vi "(SubVI) fit xyscan-data.vi"(5 "range wanted to fit":dbl, 6 "file path (dialog if empty)":path, 7 "X=T\nY=F":bool=TRUE) -> (1 "Slope (V/um)":dbl)   [LabVIEW 2014]
uses:
  <vilib>/Analysis/6fits.llb/Curve Fitting Criteria.ctl
  <vilib>/Utility/file.llb/Read From Spreadsheet File (DBL).vi
  <vilib>/Analysis/polynomials.llb/Scalar Polynomial Evaluation (DBL).vi
  <vilib>/Analysis/NI_AALPro.lvlib
panel:
  out "Radius for fit-plot":dbl[](array[numeric])
  out "Fit QPD":dbl[](array[numeric])
  out "Aligned QPD (V)":dbl[](array[numeric])
  out "Cut QPD signal (V)":dbl[](array[numeric])
  out "Cut Bead radius (nm)":dbl[](array[numeric])
  out "Bead radius (nm)":dbl[](array[numeric])
  out "Stage":dbl[](array[numeric])
  out "QPD":dbl[](array[numeric])
  out "Polynomial Coefficients":dbl[](array[numeric])
  out "XY Graph":cluster{"all rows":dbl[], "all rows":dbl[]}[](graph)
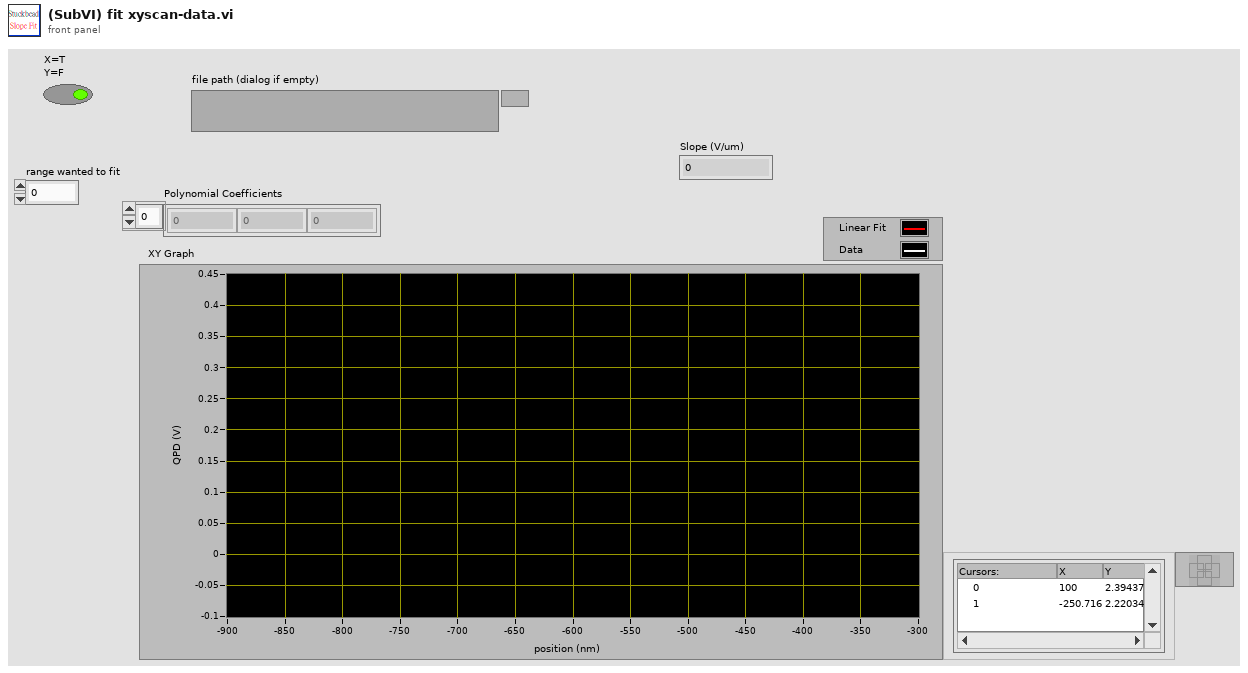
[diagram p1: front panel]
types:
  T1 = typedef "NI_AALPro.lvlib/Curve Fitting Criteria.ctl" = u16
  T2 = cluster{"Bead radius (nm)":dbl[], "Aligned QPD (V)":dbl[]}
  T3 = cluster{"Bead radius (nm)":dbl[], "Aligned QPD (V)":dbl[]}[]
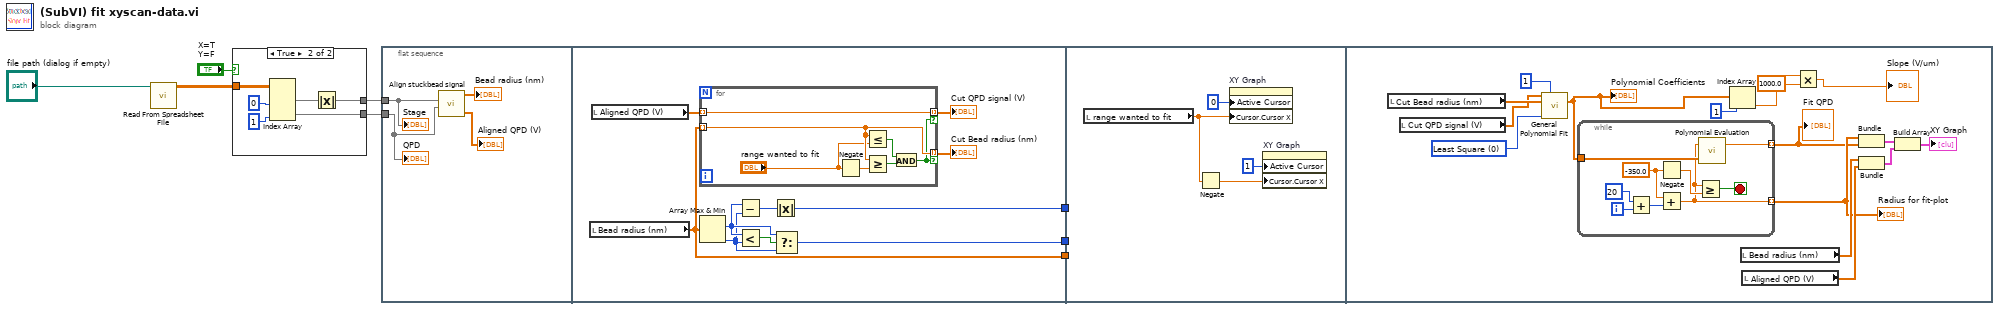
[diagram p0: block diagram]
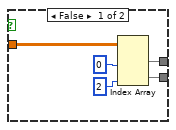
[diagram p2: hidden frame]
diagram:
  n1 = call-poly <vilib>:"Read From Spreadsheet File.vi"("file path (dialog if empty)"="file path (dialog if empty)") -> ("all rows"=w8:dbl[][])  [unwired: 6 in, 4 out]
  n2 = case shown="True" "X=T\nY=F" {
    tunnel: w8 -> [w11 w19]
    tunnel: [w10 w14] -> w6
    tunnel: [w9 w16] -> w5
    frame False {
      n3 = Index Array(array=w11, index (col) #1=0 ("disabled index (col)"), index (col) #2=2 ("index (col)")) -> (element #1=w10:dbl[], element #2=w9:dbl[])  [unwired: 2 in]
    }
    frame True {
      n4 = Index Array(array=w19, index (col) #1=0 ("disabled index (col)"), index (col) #2=1 ("index (col)")) -> (element #1=w15:dbl[], element #2=w16:dbl[])  [unwired: 2 in]
      n5 = Absolute Value(x=w15) -> (abs(x)=w14:dbl[])
    }
  }
  n6 = flat-sequence {
    tunnel: w5 -> [w22]
    tunnel: w6 -> [w23]
    tunnel: [w26] -> w4
    tunnel: [w32] -> w3
    tunnel: [w28] -> w2
    tunnel: w4 -> [_]
    tunnel: w3 -> [_]
    tunnel: w2 -> [_]
    frame #0 {
      n7 = call "Align stuckbead signal.vi"("stuckbstuck QPD (V)"=w22, "Stage (um)"=w23) -> ("Aligned QPD (V)"=→"Aligned QPD (V)":dbl[], "Bead radius (nm)"=→"Bead radius (nm)":dbl[])  [unwired: 3 in]
      "Stage" <- w23
      "QPD" <- w22
    }
    frame #1 {
      n8 = local read "Bead radius (nm)"() -> (w26:dbl[])
      n9 = local read "Aligned QPD (V)"() -> (w27:dbl[])
      n10 = for {
        tunnel: w27 -> [w40] mode=indexing
        tunnel: [w40] -> w24 mode=indexing if=w34
        tunnel: w26 -> [w38] mode=indexing
        tunnel: [w38] -> w25 mode=indexing if=w34
        n11 = Negate(x="range wanted to fit") -> (-x=w39:dbl)
        n12 = Less Or Equal?(x=w38, y="range wanted to fit") -> (x <= y?=w36:bool)
        n13 = Greater Or Equal?(x=w38, y=w39) -> (x >= y?=w35:bool)
        n14 = And(x=w36, y=w35) -> (x .and. y?=w34:bool)
      }
      "Cut Bead radius (nm)" <- w25
      "Cut QPD signal (V)" <- w24
      n15 = Array Max & Min(array=w26) -> (max index (indices)=w30:i32, min index (indices)=w29:i32)  [unwired: 2 out]
      n16 = Subtract(x=w30, y=w29) -> (x-y=w33:i32)
      n17 = Less?(x=w30, y=w29) -> (x < y?=w31:bool)
      n18 = Absolute Value(x=w33) -> (abs(x)=w32:i32)
      n19 = Select(t=w30, s=w31, f=w29) -> (s? t:f=w28:i32)
    }
    frame #2 {
      n20 = local read "range wanted to fit"() -> (w42:dbl)
      n21 = Negate(x=w42) -> (-x=w41:dbl)
      n22 = property on="XY Graph" class="XYGraph (strict)"("Active Cursor"=u32 0, "Cursor.Cursor X"=w42) -> ()  [unwired: 2 in, 2 out]
      n23 = property on="XY Graph" class="XYGraph (strict)"("Active Cursor"=u32 1, "Cursor.Cursor X"=w41) -> ()  [unwired: 2 in, 2 out]
    }
    frame #3 {
      w56 = T1 0 items=["Least Square", "Least Absolute Residual", "Bisquare"] ("method")
      n24 = local read "Cut Bead radius (nm)"() -> (w59:dbl[])
      n25 = local read "Cut QPD signal (V)"() -> (w50:dbl[])
      n26 = call <vilib>:"General Polynomial Fit.vi"("Y"=w50, "polynomial order"=1, "X"=w59, "method"=w56) -> ("Polynomial Coefficients"=w49:dbl[])  [unwired: 8 in, 3 out]
      "Polynomial Coefficients" <- w49
      n27 = while {
        tunnel: w49 -> [w69]
        tunnel: [w65] -> w51 mode=indexing
        tunnel: [w61] -> w52 mode=indexing
        i -> [w68]
        stop <- w62 stop-if-true
        w64 = -350.0
        n28 = Add(x=20, y=w68) -> (x+y=w66:i32)
        n29 = Negate(x=w64) -> (-x=w63:dbl)
        n30 = Add(x=w64, y=w66) -> (x+y=w61:dbl)
        n31 = Greater Or Equal?(x=w61, y=w63) -> (x >= y?=w62:bool)
        n32 = call-poly <vilib>:"Polynomial Evaluation.vi"("P(x)"=w69, "a"=w61) -> ("P(a)"=w65:dbl)  [unwired: 1 out]
      }
      "Fit QPD" <- w51
      "Radius for fit-plot" <- w52
      n33 = Index Array(array=w49, index=1) -> (element=w47:dbl)
      n34 = local read "Bead radius (nm)"() -> (w58:dbl[])
      n35 = local read "Aligned QPD (V)"() -> (w57:dbl[])
      n36 = Multiply(x=w47, y=1000.0) -> (x*y=→"Slope (V/um)":dbl)
      n37 = Bundle(w52, w51) -> (w60:cluster{dbl[], dbl[]})  [unwired: 1 in]
      n38 = Bundle("Bead radius (nm)"=w58, "Aligned QPD (V)"=w57) -> (w54:T2)  [unwired: 1 in]
      n39 = Build Array(w60, w54) -> (→"XY Graph":T3)
    }
  }
